vi "RTS Get Asyncronous TDMS Data.vi"(0 "File Location":path, 2 "CVS Data Input":T1 {"Station 1" format="%.6f"; "Station 2" format="%.6f"; "Station 3" format="%.6f"; "Station 4" format="%.6f"; "Station 5" format="%.6f"; "Station 6" format="%.6f"; "Station 7" format="%.6f"; "Station 8" format="%.6f"}, 5 "error in (no error)":errorcluster, 9 "Full Item Names":string[](array[string]), 11 "Station ID":string, 13 "Index Locations":i32[](array[numeric])) -> (16 "CVS Data Output":T1 {"Station 1" format="%.6f"; "Station 2" format="%.6f"; "Station 3" format="%.6f"; "Station 4" format="%.6f"; "Station 5" format="%.6f"; "Station 6" format="%.6f"; "Station 7" format="%.6f"; "Station 8" format="%.6f"}, 19 "error out":errorcluster)   [LabVIEW 2016]
uses:
  Type Definitions/RTS TDMS Data.ctl
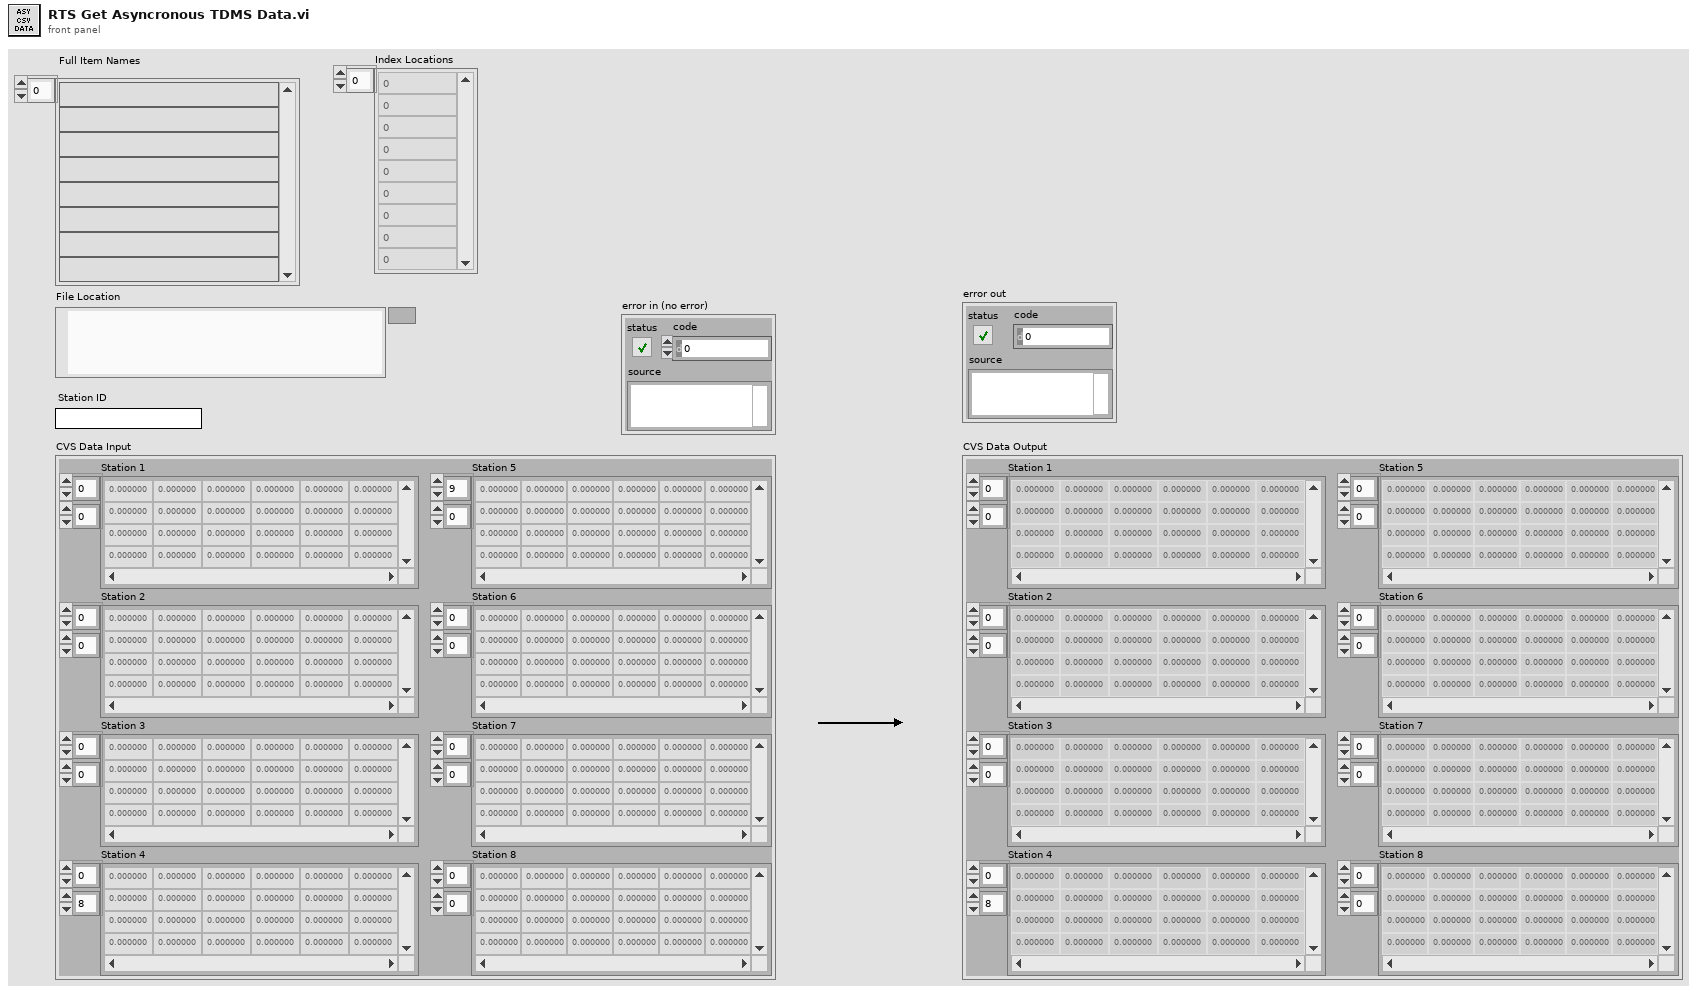
[diagram p1: front panel]
types:
  T1 = typedef "RTS TDMS Data.ctl" = cluster{"Station 1":dbl[][], "Station 2":dbl[][], "Station 3":dbl[][], "Station 4":dbl[][], "Station 5":dbl[][], "Station 6":dbl[][], "Station 7":dbl[][], "Station 8":dbl[][]}
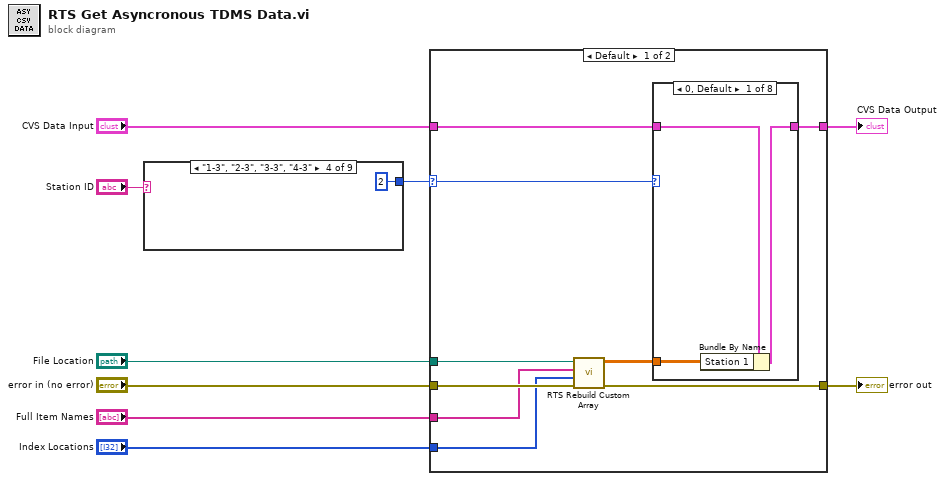
[diagram p0: block diagram]
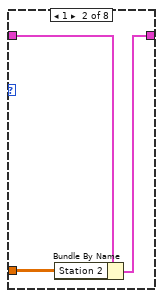
[diagram p2: hidden frame]
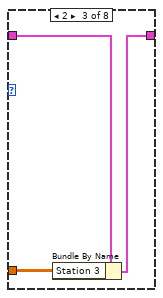
[diagram p3: hidden frame]
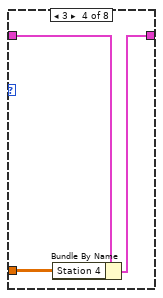
[diagram p4: hidden frame]
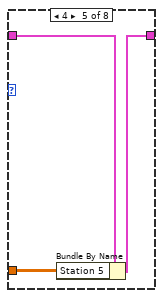
[diagram p5: hidden frame]
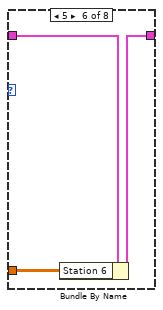
[diagram p6: hidden frame]
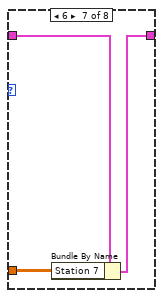
[diagram p7: hidden frame]
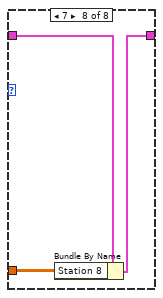
[diagram p8: hidden frame]
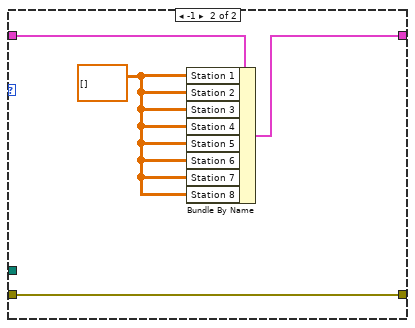
[diagram p9: hidden frame]
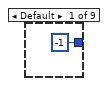
[diagram p10: hidden frame]
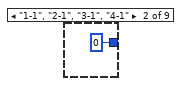
[diagram p11: hidden frame]
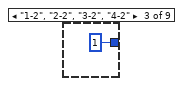
[diagram p12: hidden frame]
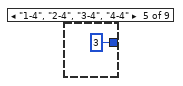
[diagram p13: hidden frame]
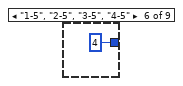
[diagram p14: hidden frame]
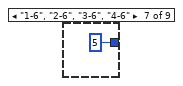
[diagram p15: hidden frame]
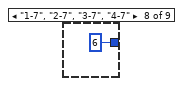
[diagram p16: hidden frame]
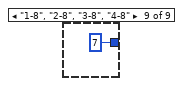
[diagram p17: hidden frame]
diagram:
  n1 = case shown="\"1-3\", \"2-3\", \"3-3\", \"4-3\"" "Station ID" {
    tunnel: [-1 ("Group Index") 0 ("Group Index") 1 ("Group Index") 2 ("Group Index") 3 ("Group Index") 4 ("Group Index") 5 ("Group Index") 6 ("Group Index") 7 ("Group Index")] -> w4
    frame Default {
    }
    frame "1-1", "2-1", "3-1", "4-1" {
    }
    frame "1-2", "2-2", "3-2", "4-2" {
    }
    frame "1-3", "2-3", "3-3", "4-3" {
    }
    frame "1-4", "2-4", "3-4", "4-4" {
    }
    frame "1-5", "2-5", "3-5", "4-5" {
    }
    frame "1-6", "2-6", "3-6", "4-6" {
    }
    frame "1-7", "2-7", "3-7", "4-7" {
    }
    frame "1-8", "2-8", "3-8", "4-8" {
    }
  }
  n2 = case shown="Default" w4 {
    selector: w4 -> [w25 _]
    tunnel: "CVS Data Input" -> [w27 w54]
    tunnel: [w26 w52] -> w8
    tunnel: [w20 w55] -> w6
    tunnel: "error in (no error)" -> [w24 w55]
    tunnel: "File Location" -> [w23 _]
    tunnel: "Full Item Names" -> [w22 _]
    tunnel: "Index Locations" -> [w21 _]
    frame Default {
      n3 = call "RTS Rebuild Custom Array.vi"("Error In"=w24, "Index Locations"=w21, "Full Item Names"=w22, "File Location"=w23) -> ("Error Out"=w20:errorcluster, "Correctly Indexed Array"=w19:dbl[][])  [unwired: 6 in]
      n4 = case shown="0, Default" w25 {
        tunnel: w27 -> [w30 w33 w36 w39 w42 w45 w48 w51]
        tunnel: [w29 w32 w35 w38 w41 w44 w47 w50] -> w26
        tunnel: w19 -> [w28 w31 w34 w37 w40 w43 w46 w49]
        frame 0, Default {
          n5 = Bundle By Name(cluster=w30, "Station 1"=w28) -> (w29:T1)
        }
        frame 1 {
          n6 = Bundle By Name(cluster=w33, "Station 2"=w31) -> (w32:T1)
        }
        frame 2 {
          n7 = Bundle By Name(cluster=w36, "Station 3"=w34) -> (w35:T1)
        }
        frame 3 {
          n8 = Bundle By Name(cluster=w39, "Station 4"=w37) -> (w38:T1)
        }
        frame 4 {
          n9 = Bundle By Name(cluster=w42, "Station 5"=w40) -> (w41:T1)
        }
        frame 5 {
          n10 = Bundle By Name(cluster=w45, "Station 6"=w43) -> (w44:T1)
        }
        frame 6 {
          n11 = Bundle By Name(cluster=w48, "Station 7"=w46) -> (w47:T1)
        }
        frame 7 {
          n12 = Bundle By Name(cluster=w51, "Station 8"=w49) -> (w50:T1)
        }
      }
    }
    frame -1 {
      w53 = dbl[][] [] ("Station 1")
      n13 = Bundle By Name(cluster=w54, "Station 1"=w53, "Station 2"=w53, "Station 3"=w53, "Station 4"=w53, "Station 5"=w53, "Station 6"=w53, "Station 7"=w53, "Station 8"=w53) -> (w52:T1)
    }
  }
  "CVS Data Output" <- w8
  "error out" <- w6
